vi "Init Msg Input.vi"(6 "Teller":refnum<class "Teller.lvclass">, 9 "Error":errorcluster, 10 "Actor":refnum<class "Actor.lvclass">) -> (2 "Msg Input":refnum<class "Msg Input.lvclass">)   [LabVIEW 2025, in "jettl.lvlib" / "Stopped jettl Msg.lvlib" / "Stopped Msg Input.lvlib"]
uses:
  Stopped Msg Input.lvlib
  Msg Input/Msg Input.lvclass
  Teller/Teller.lvclass
  Actor/Actor.lvclass
  Stopped Msg Input/Stopped Msg Input.lvclass/Stopped Msg Input.ctl
  Stopped Msg Input/Stopped Msg Input.lvclass
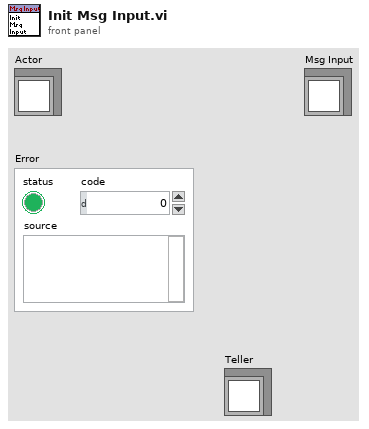
[diagram p1: front panel]
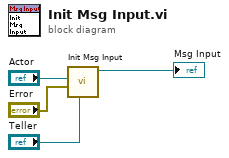
[diagram p0: block diagram]
diagram:
  n1 = call "Init Msg Input.vi"("Teller"="Teller", "Error"="Error", "Actor"="Actor") -> ("Stopped Msg Input out"=→"Msg Input":refnum<class "Stopped Msg Input.lvclass">)  [unwired: 8 in]
